vi "Globals.vi"() -> ()   [LabVIEW 2017, in "GP22_TDC_Arduinoed.lvlib"]
uses:
  GP22_TDC_Arduinoed.lvlib
  Registers.ctl
panel:
  out "Latest correction factor":dbl=1.0 format="%^#_6g"
  out "GP22 Current Registers":T1={"Reg0"=572942348, "Reg1"=557973519, "Reg2"=2684354570, "Reg3"=402653195, "Reg4"=536870913, "Reg5"=2, "Reg6"=3} {"Reg1" format="0x%08x"; "Reg2" format="0x%08x"; "Reg3" format="0x%08x"; "Reg4" format="0x%08x"; "Reg5" format="0x%08x"; "Reg0" format="0x%08x"; "Reg6" format="0x%08x"}
  out "Latest HF clock freq / Hz":dbl=4000000.0 format="%^#_6g"
  out "Latest LSB calibration / s":dbl=9e-11 format="%^#_4g"
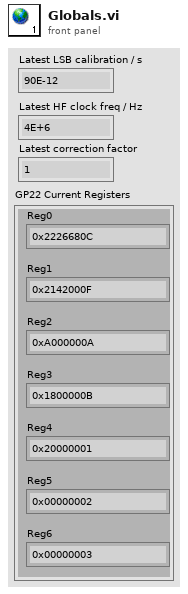
[diagram p1: front panel]
types:
  T1 = typedef "Registers.ctl" = cluster{"Reg0":u32, "Reg1":u32, "Reg2":u32, "Reg3":u32, "Reg4":u32, "Reg5":u32, "Reg6":u32}
diagram:
